vi "Translate_DBLs.vi"(7 "Translation Type":T1, 8 "error in (no error)":errorcluster, 9 "Y (North)":dbl, 10 "X (East)":dbl, 11 "CartesianVector in":refnum<class "CartesianVector.lvclass">) -> (0 "error out":errorcluster, 3 "CartesianVector out":refnum<class "CartesianVector.lvclass">)   [LabVIEW 2011, in "CartesianVector.lvclass"]
doc: "This either additively or subtractively translates a vector CV1 by the components X (East) and Y (North) and outputs it as a new Cartesian Vector. Translation type is used to select which type of translation is executed."
uses:
  CartesianVector.lvclass
  TypeDefs/TranslationType.ctl
  CartesianVector.lvclass/CartesianVector.ctl
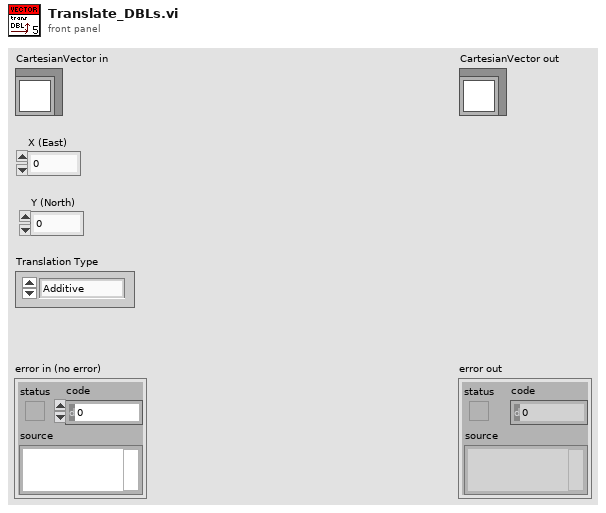
[diagram p1: front panel]
types:
  T1 = typedef "TranslationType.ctl" = enum16{"Additive", "Subtractive"}
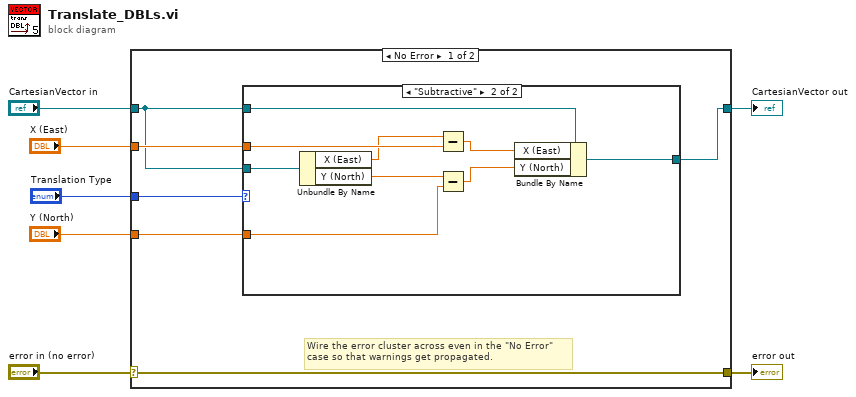
[diagram p0: block diagram]
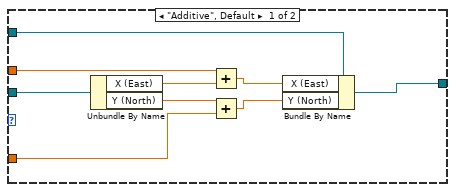
[diagram p2: hidden frame]
diagram:
  n1 = case shown="No Error" "error in (no error)" {
    selector: "error in (no error)" -> [w13 w33]
    tunnel: [w13 w33] -> w6
    tunnel: [w8 w32] -> w4
    tunnel: "CartesianVector in" -> [w9 w32]
    tunnel: "X (East)" -> [w12 _]
    tunnel: "Y (North)" -> [w11 _]
    tunnel: "Translation Type" -> [w10 _]
    frame No Error {
      # "Wire the error cluster across even in the \"No Error\"\ncase so that warnings get propagated."
      n2 = case shown="\"Subtractive\"" w10 {
        tunnel: w9 -> [w22 w31]
        tunnel: w12 -> [w18 w29]
        tunnel: w11 -> [w21 w27]
        tunnel: w9 -> [w17 w26]
        tunnel: [w15 w23] -> w8
        frame "Additive", Default {
          n3 = Unbundle By Name(w22) -> ("X (East)"=w20:dbl, "Y (North)"=w19:dbl)
          n4 = Add(x=w18, y=w20) -> (x+y=w14:dbl)
          n5 = Add(x=w19, y=w21) -> (x+y=w16:dbl)
          n6 = Bundle By Name(cluster=w17, "X (East)"=w14, "Y (North)"=w16) -> (w15:refnum<class "CartesianVector.lvclass">)
        }
        frame "Subtractive" {
          n7 = Unbundle By Name(w31) -> ("X (East)"=w28:dbl, "Y (North)"=w30:dbl)
          n8 = Subtract(x=w28, y=w29) -> (x-y=w25:dbl)
          n9 = Subtract(x=w30, y=w27) -> (x-y=w24:dbl)
          n10 = Bundle By Name(cluster=w26, "X (East)"=w25, "Y (North)"=w24) -> (w23:refnum<class "CartesianVector.lvclass">)
        }
      }
    }
    frame Error {
    }
  }
  "error out" <- w6
  "CartesianVector out" <- w4
